vi "ucgenalanSub.vi"(9 "Numeric 3":dbl, 10 "Numeric 2":dbl, 11 "Numeric":dbl) -> (3 "Numeric 4":dbl)   [LabVIEW 2024]
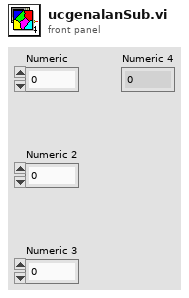
[diagram p1: front panel]
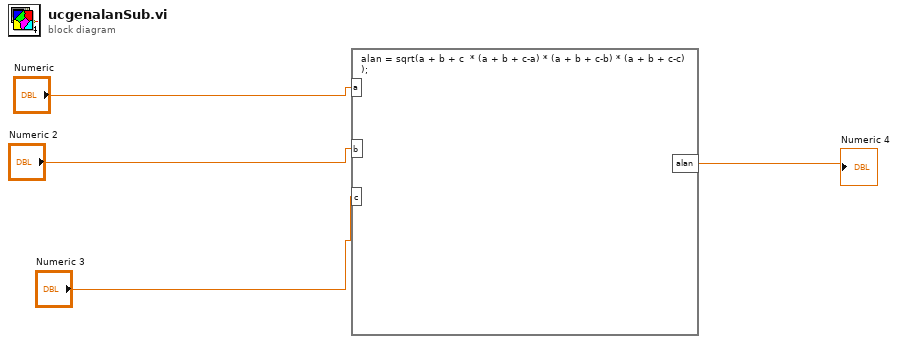
[diagram p0: block diagram]
diagram:
  n1 = formula code="alan = sqrt(a + b + c  * (a + b + c-a) * (a + b + c-b) * (a + b + c-c) );"("a"="Numeric", "b"="Numeric 2", "c"="Numeric 3") -> ("alan"=→"Numeric 4":dbl)
